vi "Error Message.vi"(0 "Error Code":i32, 11 "error in (no error)":errorcluster, 13 "ReadError?F:T":bool) -> (3 "Error Found?":bool, 4 "Error Message":string, 15 "error out":errorcluster)   [LabVIEW 2024]
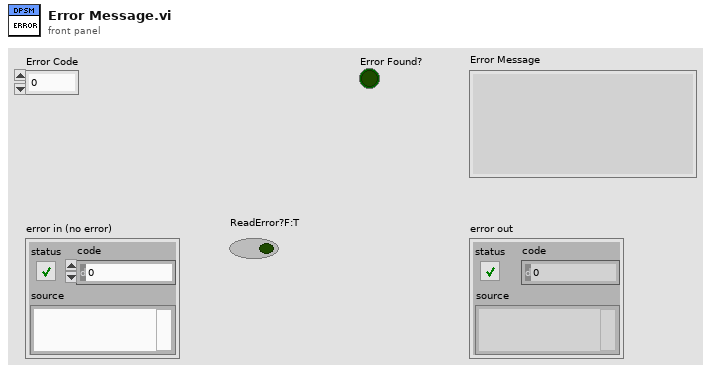
[diagram p1: front panel]
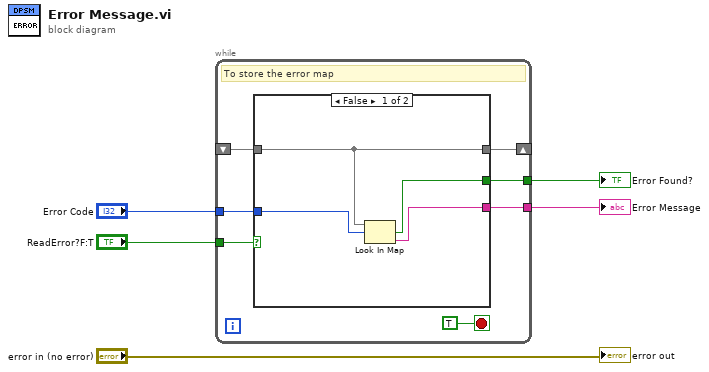
[diagram p0: block diagram]
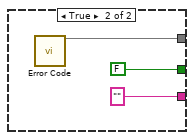
[diagram p2: hidden frame]
diagram:
  n1 = while {
    tunnel: "ReadError?F:T" -> [w12]
    shift-right: [w11] -> _
    shift-left: _ -> [w10]
    tunnel: "Error Code" -> [w9]
    tunnel: [w8] -> w3
    tunnel: [w6] -> w1
    stop <- TRUE stop-if-true
    # "To store the error map"
    n2 = case shown="False" w12 {
      tunnel: [w14 w19] -> w11
      tunnel: w10 -> [w14 _]
      tunnel: w9 -> [w16 _]
      tunnel: [w15 "" ("error message (\"\")")] -> w8
      tunnel: [w13 FALSE ("key not found?")] -> w6
      frame False {
        n3 = Look In Map(map=w14, key=w16) -> (key not found?=w13:bool, value=w15:string)  [unwired: 1 in]
      }
      frame True {
        n4 = call "Error Code.vi"() -> ("Error Map"=w19:map{i32, string})  [unwired: 15 in]
      }
    }
  }
  "Error Found?" <- w1
  "Error Message" <- w3
  "error out" <- "error in (no error)"
